vi "ScopeDownloadDSP.vi"(8 "error in (no error)":errorcluster) -> (0 "error out":errorcluster, 3 "return type":i32)   [LabVIEW 2015]
doc: "ScopeDownloadDSP\n\nDescription: \nCall this function to download the firmware file to the DSP.\nDetail: \nint ScopeDownloadDSP (\nvoid\n); \n\nParameters:\nNone\n\nReturn Values:\nA returned value of 0 indicates success. A non-zero return code will indicate error."
uses:
  ScannerDiagDLL.dll
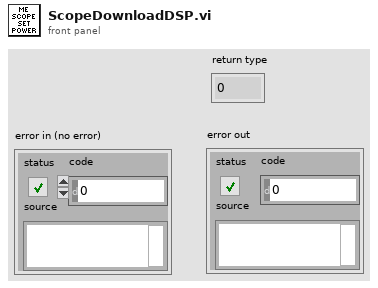
[diagram p1: front panel]
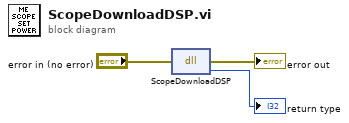
[diagram p0: block diagram]
diagram:
  n1 = dll-call lib="C:/ModisEdge/Scope/Test Sequence/Code Modules/DLL/ScannerDiagDLL.dll" fn="ScopeDownloadDSP"(error in="error in (no error)") -> (error out=→"error out":errorcluster, "return type"=→"return type":i32)  [unwired: 2 in, 1 out]
